vi "Apend System-out to Test Case Element.vi"(8 "error in (no error)":errorcluster, 9 "Result String":string, 10 "Test Case Element in":refnum<k20>, 11 "XML Report In":refnum<class "XML Report.lvclass">) -> (0 "error out":errorcluster, 2 "Test Case Element out":refnum<k20>, 3 "XML Report Out":refnum<class "XML Report.lvclass">)   [LabVIEW 2020, in "XML Report.lvclass"]
uses:
  XML Report.lvclass
  XML Report.lvclass/XML Report.ctl
  <vilib>/xml/Close Reference(Node).vi
  <resource>/objmgr/DOMUserDefRef.rc
  <vilib>/xml/NI_XML.lvlib
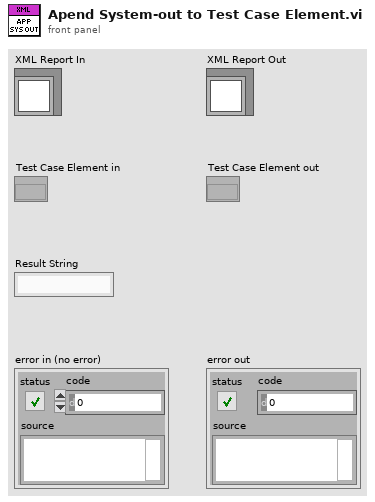
[diagram p1: front panel]
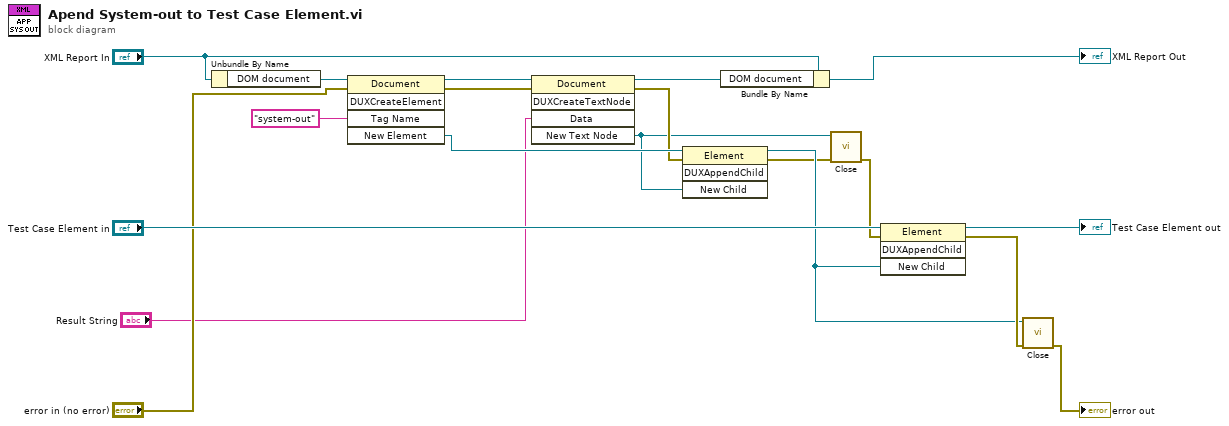
[diagram p0: block diagram]
diagram:
  n1 = Unbundle By Name("XML Report In") -> ("DOM document"=w16:refnum<k20>)
  n2 = invoke class="Document" method="DUXCreateElement"(reference=w16, error in="error in (no error)", "Tag Name"="system-out") -> (reference out=w9:refnum<k20>, error out=w7:errorcluster, "New Element"=w11:refnum<k20>)  [unwired: 2 in, 2 out]
  n3 = invoke class="Document" method="DUXCreateTextNode"(reference=w9, error in=w7, "Data"="Result String") -> (reference out=w8:refnum<k20>, error out=w6:errorcluster, "New Text Node"=w3:refnum<k20>)  [unwired: 2 in, 2 out]
  n4 = invoke class="Element" method="DUXAppendChild"(reference=w11, error in=w6, "New Child"=w3) -> (reference out=w10:refnum<k20>, error out=w5:errorcluster)  [unwired: 1 in, 2 out]
  n5 = Bundle By Name(cluster="XML Report In", "DOM document"=w8) -> (→"XML Report Out":refnum<class "XML Report.lvclass">)
  n6 = call-poly <vilib>:"Close.vi"("error in (no error)"=w5, "node"=w3) -> ("error out"=w4:errorcluster)  [unwired: 7 in]
  n7 = invoke class="Element" method="DUXAppendChild"(reference="Test Case Element in", error in=w4, "New Child"=w10) -> (reference out=→"Test Case Element out":refnum<k20>, error out=w13:errorcluster)  [unwired: 1 in, 2 out]
  n8 = call-poly <vilib>:"Close.vi"("error in (no error)"=w13, "node"=w10) -> ("error out"=→"error out":errorcluster)  [unwired: 7 in]
